vi "Auto_Routine_Swerve2Piece.vi"(8 "error in (no error)":errorcluster) -> (0 "error out":errorcluster)   [LabVIEW 2020]
uses:
  Arm/ArmPositionPreset.ctl
  Arm/ArmGamePiecePreset.ctl
  TrajectoryOrientation.ctl
  <vilib>/Rock Robotics/WPI/ThirdParty/JAS_Junk/TrajLib/Trajectory_Library.lvlib
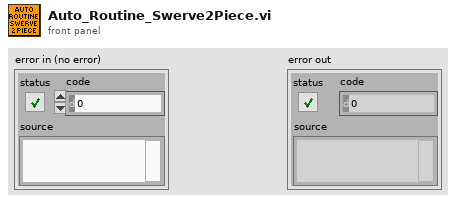
[diagram p1: front panel]
types:
  T1 = typedef "ArmGamePiecePreset.ctl" = enum16{"Cube", "Cone"}
  T2 = typedef "ArmPositionPreset.ctl" = enum16{"Upper", "Lower", "Middle", "Home", "Shelf", "Floor", "HalfFloor", "HalfHome"}
  T3 = typedef "TrajectoryOrientation.ctl" = enum16{"SameOrientation", "RotateToEndOrientation"}
  T4 = typedef "Trajectory_Library.lvlib/TRAJECTORY.ctl" = cluster{"TotalTImeSecs":dbl, "States":T5[]}
  T5 = typedef "Trajectory_Library.lvlib/TRAJ_STATE.ctl" = cluster{"TimeSeconds":dbl, "Velocity":dbl, "Acceleration":dbl, "POSE":T6, "Curvature":dbl}
  T6 = typedef "Trajectory_Library.lvlib/POSE2D.ctl" = cluster{"TRANSLATION":T7, "ROTATION":T8}
  T7 = typedef "Trajectory_Library.lvlib/TRANSLATION2D.ctl" = cluster{"X":dbl, "Y":dbl}
  T8 = typedef "Trajectory_Library.lvlib/ROTATION2D.ctl" = cluster{"VALUE":dbl, "COS":dbl, "SIN":dbl}
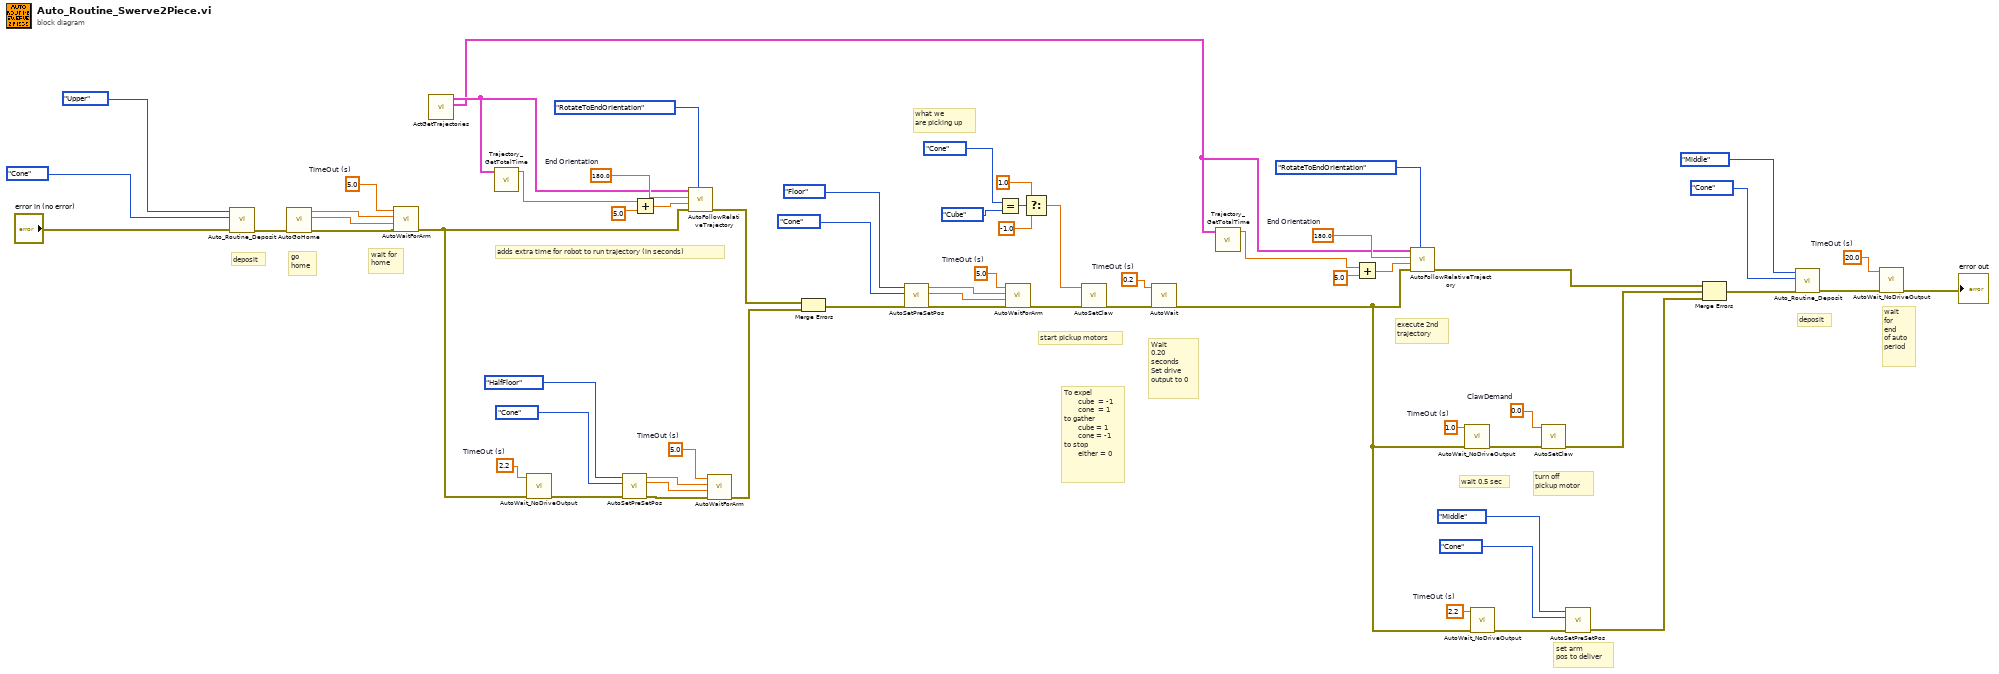
[diagram p0: block diagram]
diagram:
  w3 = 20.0  # TimeOut (s)
  w12 = 2.2  # TimeOut (s)
  w15 = 0.0  # ClawDemand
  w17 = 1.0  # TimeOut (s)
  w20 = 180.0  # End Orientation
  w32 = 0.2  # TimeOut (s)
  w39 = 2.2  # TimeOut (s)
  w47 = 5.0  # TimeOut (s)
  w53 = 5.0  # TimeOut (s)
  w56 = 180.0  # End Orientation
  w61 = 5.0  # TimeOut (s)
  # "wait\nfor \nend\nof auto\nperiod"
  # "deposit"
  # "what we\nare picking up"
  # "Wait\n0.20\nseconds\nSet drive\noutput to 0"
  # "To expel\n       cube  = -1\n       cone  = 1\nto gather\n       cube = 1\n       cone = -1\nto stop\n       either = 0"
  # "wait for\nhome"
  # "go\nhome"
  # "deposit"
  # "set arm\npos to deliver"
  # "turn off\npickup motor"
  # "wait 0.5 sec"
  # "execute 2nd\ntrajectory"
  # "start pickup motors"
  # "adds extra time for robot to run trajectory (in seconds)"
  n1 = call "Auto_Routine_Deposit.vi"("error in (no error)"="error in (no error)", "Game Piece"=ArmGamePiecePreset."Cone", "Position"=ArmPositionPreset."Upper") -> ("error out"=w60:errorcluster)  [unwired: 8 in]
  n2 = call "AutoGoHome.vi"("error in (no error)"=w60) -> ("error out"=w42:errorcluster, "Desired Extend"=w40:dbl, "Desired Lift"=w41:dbl)  [unwired: 8 in]
  n3 = call "AutoWaitForArm.vi"("error in (no error)"=w42, "Desired Extend"=w40, "Desired Lift"=w41, "TimeOut (s)"=w61) -> ("error out"=w38:errorcluster)  [unwired: 7 in]
  n4 = call "ActGetTrajectories.vi"() -> ("Trajectory2"=w18:T4, "Trajectory1"=w55:T4)  [unwired: 8 in, 2 out]
  n5 = call <vilib>:"Trajectory_GetTotalTime.vi"("TRAJECTORY"=w55) -> ("TotalTime_Sec"=w54:dbl)  [unwired: 10 in]
  n6 = call "AutoWait_NoDriveOutput.vi"("error in (no error)"=w38, "TimeOut (s)"=w39) -> ("error out"=w37:errorcluster)  [unwired: 9 in]
  n7 = call "AutoSetPreSetPos.vi"("error in (no error)"=w37, "Game Piece"=ArmGamePiecePreset."Cone", "Position"=ArmPositionPreset."HalfFloor") -> ("error out"=w51:errorcluster, "Desired Extend"=w35:dbl, "Desired Lift"=w36:dbl)  [unwired: 6 in]
  n8 = Add(x=w54, y=5.0) -> (x+y=w58:dbl)
  n9 = call "AutoFollowRelativeTrajectory.vi"("Orientation"=TrajectoryOrientation."RotateToEndOrientation", "error in (no error)"=w38, "TimeOut (s)"=w58, "End Orientation"=w56, "Trajectory"=w55) -> ("error out"=w49:errorcluster)  [unwired: 6 in]
  n10 = call "AutoWaitForArm.vi"("error in (no error)"=w51, "Desired Extend"=w35, "Desired Lift"=w36, "TimeOut (s)"=w53) -> ("error out"=w48:errorcluster)  [unwired: 7 in]
  n11 = Merge Errors(w49, w48) -> (w43:errorcluster)
  n12 = call "AutoSetPreSetPos.vi"("error in (no error)"=w43, "Game Piece"=ArmGamePiecePreset."Cone", "Position"=ArmPositionPreset."Floor") -> ("error out"=w45:errorcluster, "Desired Extend"=w33:dbl, "Desired Lift"=w34:dbl)  [unwired: 6 in]
  n13 = Equal?(x=ArmGamePiecePreset."Cone", y=ArmGamePiecePreset."Cube") -> (x = y?=w29:bool)
  n14 = call "AutoWaitForArm.vi"("error in (no error)"=w45, "Desired Extend"=w33, "Desired Lift"=w34, "TimeOut (s)"=w47) -> ("error out"=w24:errorcluster)  [unwired: 7 in]
  n15 = Select(t=1.0, s=w29, f=-1.0) -> (s? t:f=w28:dbl)
  n16 = call "AutoSetClaw.vi"("error in (no error)"=w24, "ClawDemand"=w28) -> ("error out"=w31:errorcluster)  [unwired: 9 in]
  n17 = call "AutoWait.vi"("error in (no error)"=w31, "TimeOut (s)"=w32) -> ("error out"=w10:errorcluster)  [unwired: 9 in]
  n18 = call <vilib>:"Trajectory_GetTotalTime.vi"("TRAJECTORY"=w18) -> ("TotalTime_Sec"=w19:dbl)  [unwired: 10 in]
  n19 = Add(x=w19, y=5.0) -> (x+y=w22:dbl)
  n20 = call "AutoFollowRelativeTrajectory.vi"("Orientation"=TrajectoryOrientation."RotateToEndOrientation", "error in (no error)"=w10, "TimeOut (s)"=w22, "End Orientation"=w20, "Trajectory"=w18) -> ("error out"=w9:errorcluster)  [unwired: 6 in]
  n21 = call "AutoWait_NoDriveOutput.vi"("error in (no error)"=w10, "TimeOut (s)"=w17) -> ("error out"=w16:errorcluster)  [unwired: 9 in]
  n22 = call "AutoWait_NoDriveOutput.vi"("error in (no error)"=w10, "TimeOut (s)"=w12) -> ("error out"=w11:errorcluster)  [unwired: 9 in]
  n23 = call "AutoSetClaw.vi"("error in (no error)"=w16, "ClawDemand"=w15) -> ("error out"=w8:errorcluster)  [unwired: 9 in]
  n24 = call "AutoSetPreSetPos.vi"("error in (no error)"=w11, "Game Piece"=ArmGamePiecePreset."Cone", "Position"=ArmPositionPreset."Middle") -> ("error out"=w7:errorcluster)  [unwired: 6 in, 2 out]
  n25 = Merge Errors(w9, w8, w7) -> (w4:errorcluster)
  n26 = call "Auto_Routine_Deposit.vi"("error in (no error)"=w4, "Game Piece"=ArmGamePiecePreset."Cone", "Position"=ArmPositionPreset."Middle") -> ("error out"=w2:errorcluster)  [unwired: 8 in]
  n27 = call "AutoWait_NoDriveOutput.vi"("error in (no error)"=w2, "TimeOut (s)"=w3) -> ("error out"=→"error out":errorcluster)  [unwired: 9 in]
